vi "DestroySelfReference.vi"(8 "error in (no error)":errorcluster, 11 "Measurement.Free":refnum<class "Measurement.Free.lvclass">) -> (0 "error out":errorcluster, 3 "Measurement.Free out":refnum<class "Measurement.Free.lvclass">)   [LabVIEW 2017, in "Measurement.Free.lvclass"]
doc: "JKI State Machine Objects (SMO) 1.0.0.5\nJKI - JKI\nCopyright (c) 2016, JKI"
uses:
  Measurement.Free.lvclass
  Measurement.Free.lvclass/Measurement.Free.ctl
  Measurement/Measurement.lvclass
panel:
  # "For instructions on how to use the JKI State Machine Objects, examples and video tutorials, visit:\nhttp://jki.net/state-machine-objects/\n\nJKI State Machine Objects™\nhttp://jki.net/state-machine-objects/\nCopyright (C) 2005-2015, JKI <info@jki.net>\nALL RIGHTS RESERVED"
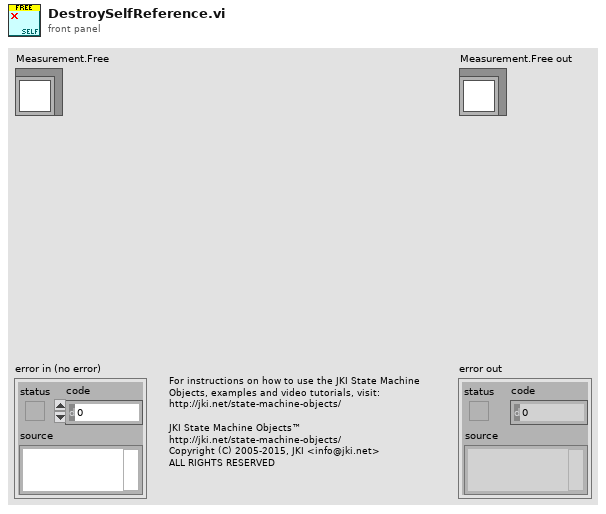
[diagram p1: front panel]
types:
  T1 = typedef "Measurement.Free.lvclass/PrivateData--Ref.ctl" = refnum<data-value>
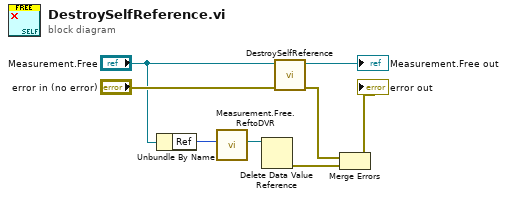
[diagram p0: block diagram]
diagram:
  n1 = Unbundle By Name("Measurement.Free") -> ("Ref"=w2:u32)
  n2 = call "Measurement.Free.ReftoDVR.vi"("Ref"=w2) -> ("Ref"=w1:T1)  [unwired: 10 in]
  n3 = Delete Data Value Reference(data value reference=w1) -> (error out=w5:errorcluster)  [unwired: 1 in, 1 out]
  n4 = call-parent "DestroySelfReference.vi"("error in (no error)"="error in (no error)", "Measurement"="Measurement.Free") -> ("error out"=w4:errorcluster, "Measurement out"=→"Measurement.Free out":refnum<class "Measurement.Free.lvclass">)  [unwired: 8 in]
  n5 = Merge Errors(w4, w5) -> (→"error out":errorcluster)
